vi "Min Read Array.vi"(8 "error in":errorcluster, 11 "Min Pressure Limit in":refnum<class "Pressure Limit.lvclass">) -> (0 "error out":errorcluster, 1 "Changed or First Call?":bool, 2 "Pressure Min SP":dbl[](array[numeric]), 3 "Min Pressure Limit out":refnum<class "Pressure Limit.lvclass">)   [LabVIEW 2023, in "Pressure Limit.lvclass"]
uses:
  Pressure Limit.lvclass
  Parents/Limit/Limit.lvclass
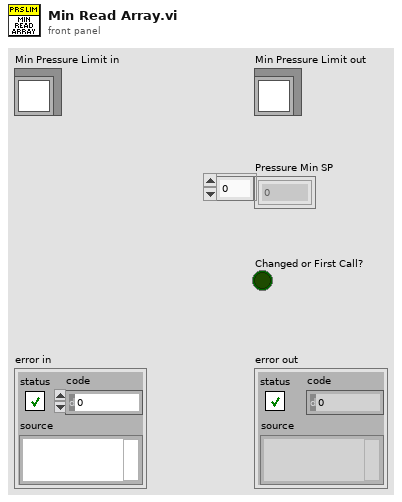
[diagram p1: front panel]
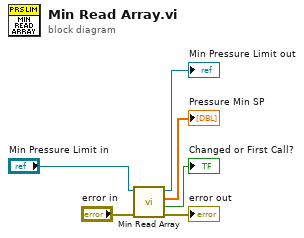
[diagram p0: block diagram]
diagram:
  n1 = call-parent "Min Read Array.vi"("error in"="error in", "Min Limit in"="Min Pressure Limit in") -> ("error out"=→"error out":errorcluster, "Changed or First Call?"=→"Changed or First Call?":bool, "Current Min SP"=→"Pressure Min SP":dbl[], "Min Limit out"=→"Min Pressure Limit out":refnum<class "Pressure Limit.lvclass">)  [unwired: 6 in]
